vi "Write threshold.vi"(8 "error in (no error)":errorcluster, 10 "Severity":T1=enum."INFO", 11 "SetGlobalThreshold in":refnum<class "SetGlobalThresholdMsg.lvclass">) -> (0 "error out":errorcluster, 3 "SetGlobalThreshold out":refnum<class "SetGlobalThresholdMsg.lvclass">)   [LabVIEW 2026, in "Lumberjack.lvlib" / "SetGlobalThresholdMsg.lvclass"]
doc: "Stores a Severity threshold into this SetGlobalThresholdMsg's private data.\nClass private-data accessor; sets the message's `threshold` field with no side effects.\nLumberjack.lvlib, SetGlobalThresholdMsg.lvclass, public."
uses:
  SetGlobalThresholdMsg.lvclass
  TypeDefs/Severity.ctl
  SetGlobalThresholdMsg.lvclass/SetGlobalThresholdMsg.ctl
  Lumberjack.lvlib
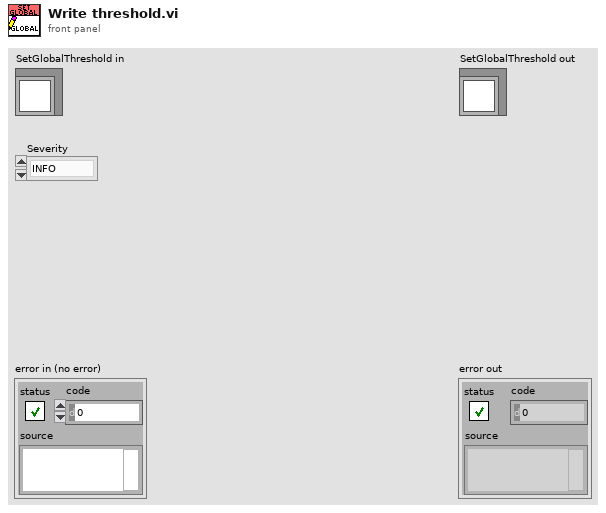
[diagram p1: front panel]
types:
  T1 = typedef "Lumberjack.lvlib/Severity.ctl" = enum16{"OFF", "FATAL", "ERROR", "WARN", "INFO", "DEBUG", "TRACE", "ALL"}
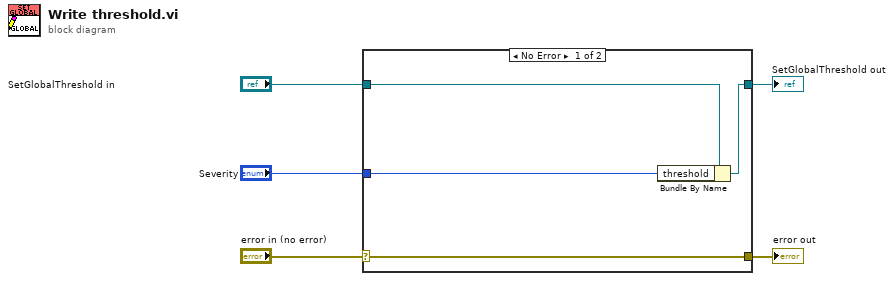
[diagram p0: block diagram]
diagram:
  n1 = case shown="No Error" "error in (no error)" {
    selector: "error in (no error)" -> [w9 w10]
    tunnel: [w9 w10] -> w4
    tunnel: [w7 w11] -> w2
    tunnel: "SetGlobalThreshold in" -> [w8 w11]
    tunnel: "Severity" -> [w6 _]
    frame No Error {
      n2 = Bundle By Name(cluster=w8, "threshold"=w6) -> (w7:refnum<class "SetGlobalThresholdMsg.lvclass">)
    }
    frame Error {
    }
  }
  "error out" <- w4
  "SetGlobalThreshold out" <- w2
